vi "Prompt for Step--Init UI.vi"(8 "error in (no error)":errorcluster, 10 "Control Ref Map":map{string, refnum<vi>}(c390), 11 "Mouse Action in":refnum<class "Mouse Action.lvclass">) -> (0 "error out":errorcluster, 3 "Mouse Action out":refnum<class "Mouse Action.lvclass">)   [LabVIEW 2020, in "MacroAssert.lvlib" / "Mouse Action.lvclass"]
uses:
  Mouse Action.lvclass
  Action Step/Action Step.lvclass
  Mouse Action.lvclass/Mouse Action.ctl
  MacroAssert.lvlib
  Support/Get Control Reference by Label (1D STR).vi
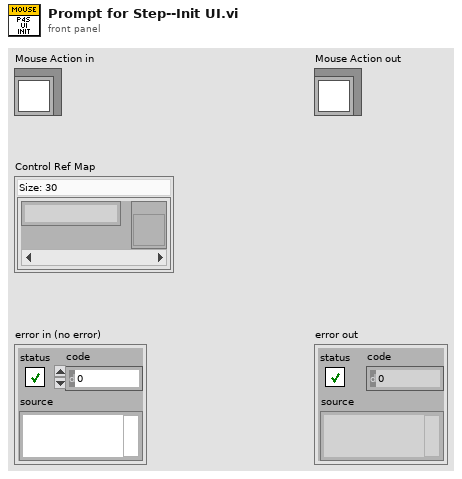
[diagram p1: front panel]
types:
  T1 = typedef "MacroAssert.lvlib/Mouse Action.lvclass/Mouse Action Type.ctl" = enum16{"Click", "Absolute Move", "Absolute Move and Click", "Relative Move", "Relative Move and Click", "Wheel Up", "Wheel Down"}
  T2 = typedef "MacroAssert.lvlib/Mouse Action.lvclass/Button.ctl" = enum16{"Left", "Right", "Middle"}
  T3 = typedef "MacroAssert.lvlib/Mouse Action.lvclass/Click Type.ctl" = enum16{"Normal", "Hold", "Release"}
  T4 = typedef "MacroAssert.lvlib/Mouse Action.lvclass/Relative Movement Type.ctl" = enum16{"Pixels from Current Position", "Pixels from Top-Left of Control", "Pixels from Top-Left of Window", "Percentage from Top-Left of Control", "Percentage from Top-Left of Window", "Percentage from Top-Left of Screen"}
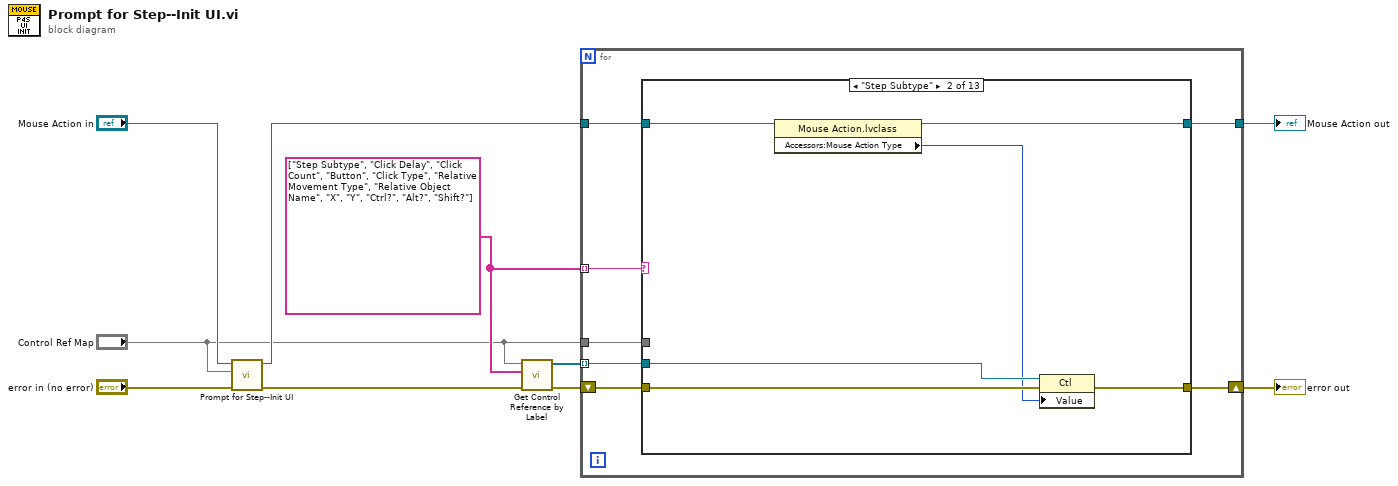
[diagram p0: block diagram]
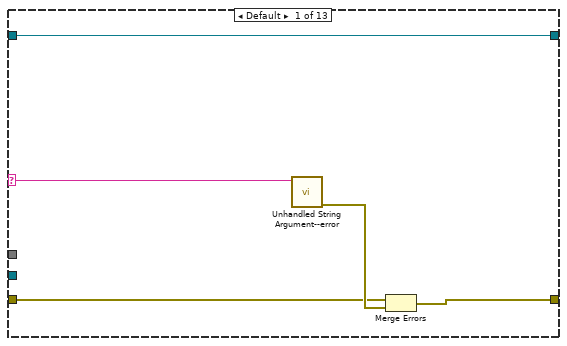
[diagram p2: hidden frame]
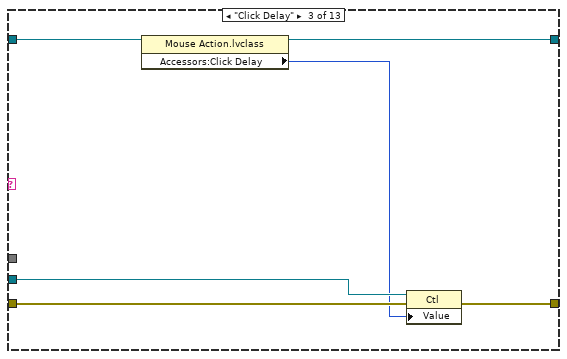
[diagram p3: hidden frame]
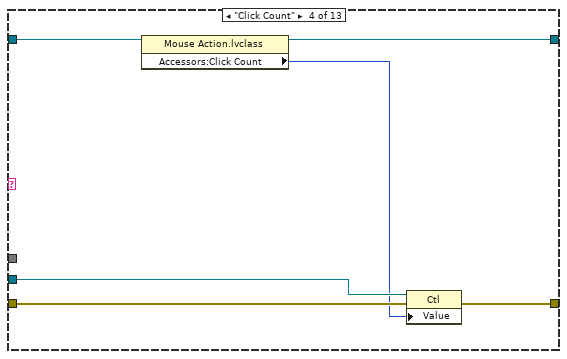
[diagram p4: hidden frame]
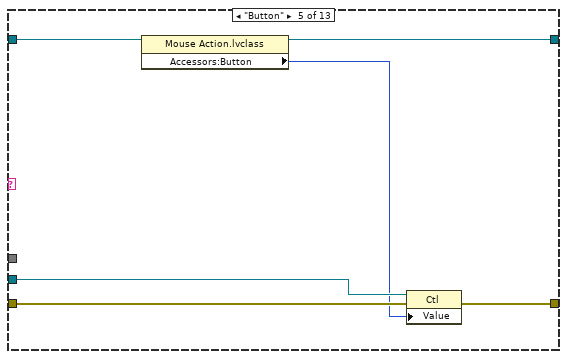
[diagram p5: hidden frame]
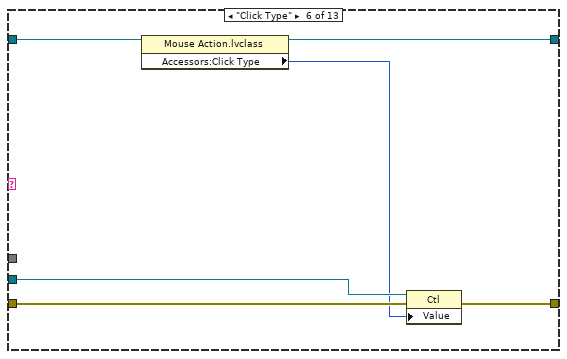
[diagram p6: hidden frame]
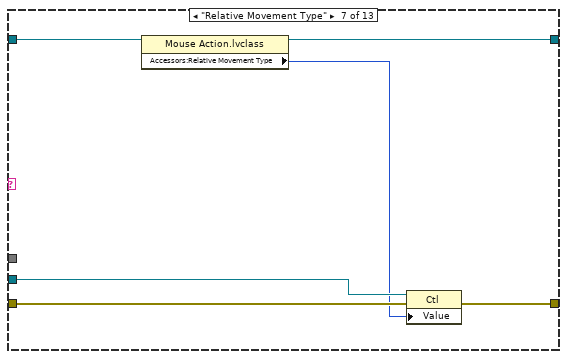
[diagram p7: hidden frame]
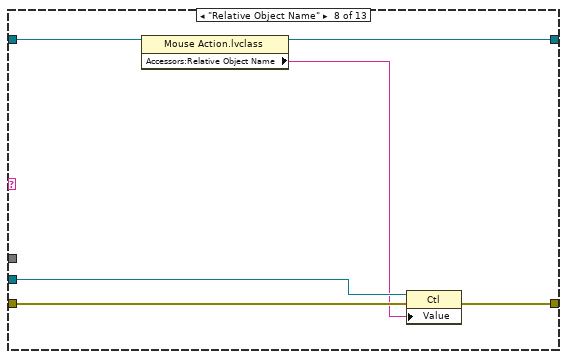
[diagram p8: hidden frame]
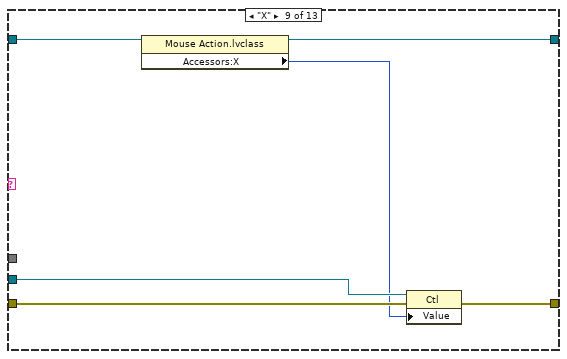
[diagram p9: hidden frame]
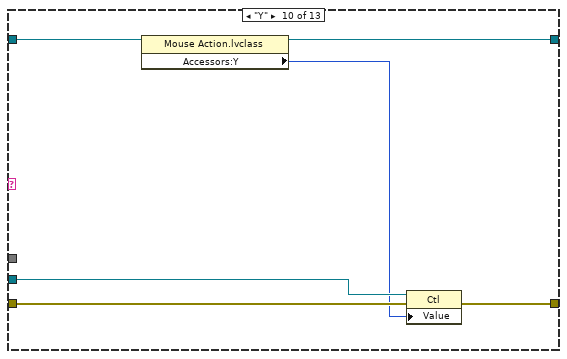
[diagram p10: hidden frame]
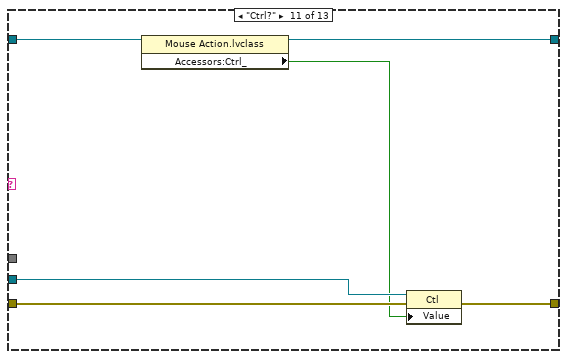
[diagram p11: hidden frame]
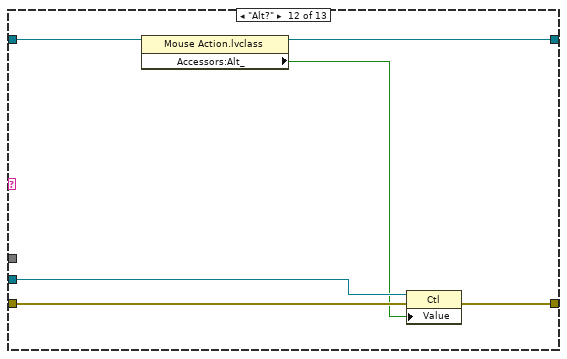
[diagram p12: hidden frame]
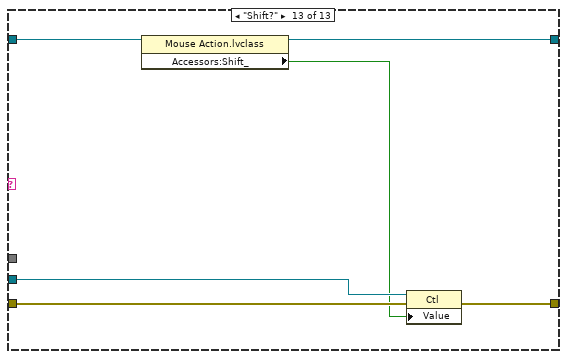
[diagram p13: hidden frame]
diagram:
  w9 = string[] ["Step Subtype", "Click Delay", "Click Count", "Button", "Click Type", "Relative Movement Type", "Relative Object Name", "X", "Y", "Ctrl?", "Alt?", "Shift?"]
  n1 = call-parent "Prompt for Step--Init UI.vi"("error in (no error)"="error in (no error)", "Control Ref Map"="Control Ref Map", "Step in"="Mouse Action in") -> ("error out"=w5:errorcluster, "Step out"=w2:refnum<class "Mouse Action.lvclass">)  [unwired: 7 in]
  n2 = call-poly "Get Control Reference by Label.vi"("error in (no error)"=w5, "Control Names"=w9, "Control Ref Map"="Control Ref Map") -> ("error out"=w10:errorcluster, "Control Refs"=w8:refnum<vi>[])  [unwired: 6 in, 1 out]
  n3 = for {
    tunnel: w2 -> [w15]
    tunnel: [w13] -> w6
    tunnel: w9 -> [w16] mode=indexing
    tunnel: w8 -> [w14] mode=indexing
    shift-right: [w12] -> w7
    shift-left: w10 -> [w17]
    tunnel: "Control Ref Map" -> [w11]
    n4 = case shown="\"Step Subtype\"" w16 {
      selector: w16 -> [w19 _ _ _ _ _ _ _ _ _ _ _ _]
      tunnel: w17 -> [w21 w25 w31 w37 w43 w49 w55 w61 w67 w73 w79 w85 w91]
      tunnel: w15 -> [w18 w28 w34 w40 w46 w52 w58 w64 w70 w76 w82 w88 w94]
      tunnel: w14 -> [_ w26 w32 w38 w44 w50 w56 w62 w68 w74 w80 w86 w92]
      tunnel: [w18 w27 w33 w39 w45 w51 w57 w63 w69 w75 w81 w87 w93] -> w13
      tunnel: [w20 w23 w29 w35 w41 w47 w53 w59 w65 w71 w77 w83 w89] -> w12
      tunnel: w11 -> [_ _ _ _ _ _ _ _ _ _ _ _ _]
      frame Default {
        n5 = call "Unhandled String Argument--error.vi"("Argument"=w19) -> ("error out"=w22:errorcluster)  [unwired: 10 in]
        n6 = Merge Errors(w21, w22) -> (w20:errorcluster)
      }
      frame "Step Subtype" {
        n7 = property class="Mouse Action.lvclass"(reference=w28) -> (reference out=w27:refnum<class "Mouse Action.lvclass">, "Accessors:Mouse Action Type"=w24:T1)  [unwired: 1 in, 1 out]
        n8 = property class="Ctl"(reference=w26, error in=w25, "Value"=w24) -> (error out=w23:errorcluster)  [unwired: 1 out]
      }
      frame "Click Delay" {
        n9 = property class="Mouse Action.lvclass"(reference=w34) -> (reference out=w33:refnum<class "Mouse Action.lvclass">, "Accessors:Click Delay"=w30:i32)  [unwired: 1 in, 1 out]
        n10 = property class="Ctl"(reference=w32, error in=w31, "Value"=w30) -> (error out=w29:errorcluster)  [unwired: 1 out]
      }
      frame "Click Count" {
        n11 = property class="Mouse Action.lvclass"(reference=w40) -> (reference out=w39:refnum<class "Mouse Action.lvclass">, "Accessors:Click Count"=w36:i32)  [unwired: 1 in, 1 out]
        n12 = property class="Ctl"(reference=w38, error in=w37, "Value"=w36) -> (error out=w35:errorcluster)  [unwired: 1 out]
      }
      frame "Button" {
        n13 = property class="Mouse Action.lvclass"(reference=w46) -> (reference out=w45:refnum<class "Mouse Action.lvclass">, "Accessors:Button"=w42:T2)  [unwired: 1 in, 1 out]
        n14 = property class="Ctl"(reference=w44, error in=w43, "Value"=w42) -> (error out=w41:errorcluster)  [unwired: 1 out]
      }
      frame "Click Type" {
        n15 = property class="Mouse Action.lvclass"(reference=w52) -> (reference out=w51:refnum<class "Mouse Action.lvclass">, "Accessors:Click Type"=w48:T3)  [unwired: 1 in, 1 out]
        n16 = property class="Ctl"(reference=w50, error in=w49, "Value"=w48) -> (error out=w47:errorcluster)  [unwired: 1 out]
      }
      frame "Relative Movement Type" {
        n17 = property class="Mouse Action.lvclass"(reference=w58) -> (reference out=w57:refnum<class "Mouse Action.lvclass">, "Accessors:Relative Movement Type"=w54:T4)  [unwired: 1 in, 1 out]
        n18 = property class="Ctl"(reference=w56, error in=w55, "Value"=w54) -> (error out=w53:errorcluster)  [unwired: 1 out]
      }
      frame "Relative Object Name" {
        n19 = property class="Mouse Action.lvclass"(reference=w64) -> (reference out=w63:refnum<class "Mouse Action.lvclass">, "Accessors:Relative Object Name"=w60:string)  [unwired: 1 in, 1 out]
        n20 = property class="Ctl"(reference=w62, error in=w61, "Value"=w60) -> (error out=w59:errorcluster)  [unwired: 1 out]
      }
      frame "X" {
        n21 = property class="Mouse Action.lvclass"(reference=w70) -> (reference out=w69:refnum<class "Mouse Action.lvclass">, "Accessors:X"=w66:i32)  [unwired: 1 in, 1 out]
        n22 = property class="Ctl"(reference=w68, error in=w67, "Value"=w66) -> (error out=w65:errorcluster)  [unwired: 1 out]
      }
      frame "Y" {
        n23 = property class="Mouse Action.lvclass"(reference=w76) -> (reference out=w75:refnum<class "Mouse Action.lvclass">, "Accessors:Y"=w72:i32)  [unwired: 1 in, 1 out]
        n24 = property class="Ctl"(reference=w74, error in=w73, "Value"=w72) -> (error out=w71:errorcluster)  [unwired: 1 out]
      }
      frame "Ctrl?" {
        n25 = property class="Mouse Action.lvclass"(reference=w82) -> (reference out=w81:refnum<class "Mouse Action.lvclass">, "Accessors:Ctrl_"=w78:bool)  [unwired: 1 in, 1 out]
        n26 = property class="Ctl"(reference=w80, error in=w79, "Value"=w78) -> (error out=w77:errorcluster)  [unwired: 1 out]
      }
      frame "Alt?" {
        n27 = property class="Mouse Action.lvclass"(reference=w88) -> (reference out=w87:refnum<class "Mouse Action.lvclass">, "Accessors:Alt_"=w84:bool)  [unwired: 1 in, 1 out]
        n28 = property class="Ctl"(reference=w86, error in=w85, "Value"=w84) -> (error out=w83:errorcluster)  [unwired: 1 out]
      }
      frame "Shift?" {
        n29 = property class="Mouse Action.lvclass"(reference=w94) -> (reference out=w93:refnum<class "Mouse Action.lvclass">, "Accessors:Shift_"=w90:bool)  [unwired: 1 in, 1 out]
        n30 = property class="Ctl"(reference=w92, error in=w91, "Value"=w90) -> (error out=w89:errorcluster)  [unwired: 1 out]
      }
    }
  }
  "error out" <- w7
  "Mouse Action out" <- w6
